vi "Drivetrain Read Encoders.vi"(6 "Reset Encoders":bool) -> (3 "Drivetrain Encoder Values":T1)   [LabVIEW 2016]
uses:
  Common Code/Drivetrain Encoder Values.ctl
  Common Code/Encoder Values.ctl
  Robot Global Data.vi
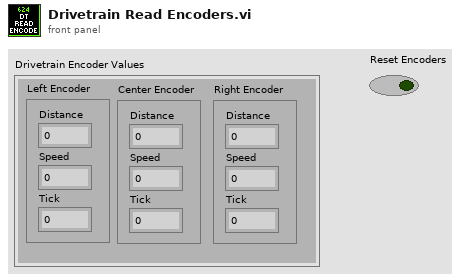
[diagram p1: front panel]
types:
  T1 = typedef "Drivetrain Encoder Values.ctl" = cluster{"Left Encoder":T2, "Center Encoder":T2, "Right Encoder":T2}
  T2 = typedef "Encoder Values.ctl" = cluster{"Distance":dbl, "Speed":dbl, "Tick":dbl}
  T3 = typedef "Dashboard Control Data.ctl" = cluster{"Drivetrain Settings":T4, "Intake Presets ":T6, "Shooter Presets":T7, "Vision Target Packet":T10, "Auton Presets":cluster{"Start Position":dbl}, "Drivetrain Encoder Values":T1, "Drivetrain Encoder Settings":cluster{"Left Tick Constant":dbl, "Right Tick Contant":dbl, "Reset Encoders":bool, "Center Tick Constant":dbl}, "Zero Gyro":bool}
  T4 = typedef "Drivetrain Settings.ctl" = cluster{"Gyro Tolerance":dbl, "Gyro Steer PID Gains":T5, "Y Power Multiplier":dbl, "Turn Power Multiplier":dbl, "Gyro Output":dbl, "Creep Rate":dbl, "Distance Drive PID Gains":T5, "Distance Tolerance":dbl, "Distance Output":dbl, "Strafe Threshold":dbl, "Strafe Correct":bool, "Strafe Corect Tolerance":dbl, "Translate Drive PID Gains":T5, "Strafe Output":dbl, "SC Right":dbl, "SC Left":dbl, "Use Gyro":bool, "Constant Power":bool, "Strafe Power":dbl}
  T5 = typedef "PID Gains.ctl" = cluster{"proportional gain (Kc)":dbl, "integral time (Ti, min)":dbl, "derivative time (Td, min)":dbl}
  T6 = typedef "Intake Presets.ctl" = cluster{"Intake Speed ":dbl, "Outake Speed":dbl, "Current Trip Delay":dbl, "Max Current":dbl}
  T7 = typedef "Shooter Presets.ctl" = cluster{"Key Shot":cluster{"RPM ":dbl, "Hood?":bool}, "Distance Shot":cluster{"RPM":dbl, "Hood?":bool}, "RPM Tolerance":dbl, "Wheel C":dbl, "Vision Shot Presets":T8, "Hopper speed":dbl, "manuel presets":T9}
  T8 = typedef "Vision Shot Presets.ctl" = cluster{"Vision Dist RPM":dbl, "Vision RPM ":dbl, "Vision Dist Hood":bool, "Vision Hood":bool, "Vision Far Dist":dbl, "is we far??":bool}
  T9 = typedef "Manual Shooter Presets.ctl" = cluster{"change delay":dbl}
  T10 = typedef "Vision Target Packet.ctl" = cluster{"Robot Center":dbl, "Center X":dbl, "Center Y":dbl, "Angle":dbl, "Distance":dbl, "Found Target?":bool}
  T11 = typedef "WPI_EncoderDevRef.ctl" = cluster{"DevStatus":errorcluster, "EncoderIndex":T12, "CounterIndex":T13, "DistancePerCount":dbl, "Decoding Type":T14}
  T12 = typedef "FPGA_EncoderIdx.ctl" = enum8{"Enc 0", "Enc 1", "Enc 2", "Enc 3", "Enc 4", "Enc 5", "Enc 6", "Enc 7", "Invalid"}
  T13 = typedef "FPGA_CounterCtrSystemIndex.ctl" = enum8{"Ctr 0", "Ctr 1", "Ctr 2", "Ctr 3", "Ctr 4", "Ctr 5", "Ctr 6", "Ctr 7", "Invalid"}
  T14 = typedef "WPI_EncoderType.ctl" = enum16{"1x", "2x", "4x"}
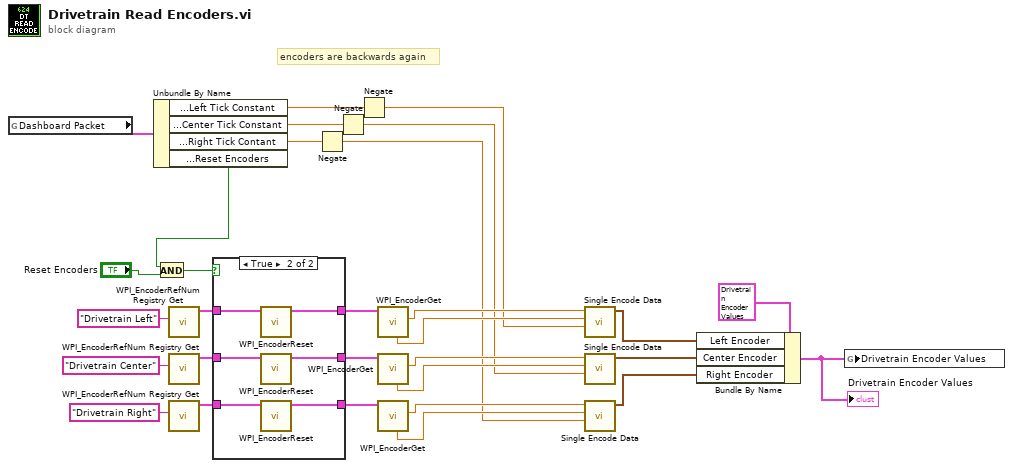
[diagram p0: block diagram]
diagram:
  # "encoders are backwards again"
  n1 = global read "Robot Global Data.vi" "Dashboard Packet"() -> (w13:T3)
  n2 = Unbundle By Name(w13) -> ("Drivetrain Encoder Settings.Left Tick Constant"=w12:dbl, "Drivetrain Encoder Settings.Center Tick Constant"=w11:dbl, "Drivetrain Encoder Settings.Right Tick Contant"=w10:dbl, "Drivetrain Encoder Settings.Reset Encoders"=w1:bool)
  n3 = And(x=w1, y="Reset Encoders") -> (x .and. y?=w2:bool)
  n4 = call <vilib>:"WPI_EncoderRefNum Registry Get.vi"("refnum name"="Drivetrain Left") -> ("EncoderDevRef"=w30:T11)  [unwired: 9 in, 1 out]
  n5 = call <vilib>:"WPI_EncoderRefNum Registry Get.vi"("refnum name"="Drivetrain Center") -> ("EncoderDevRef"=w29:T11)  [unwired: 9 in, 1 out]
  n6 = call <vilib>:"WPI_EncoderRefNum Registry Get.vi"("refnum name"="Drivetrain Right") -> ("EncoderDevRef"=w27:T11)  [unwired: 9 in, 1 out]
  n7 = case shown="True" w2 {
    tunnel: w30 -> [w33 w39]
    tunnel: w29 -> [w32 w38]
    tunnel: w27 -> [w31 w37]
    tunnel: [w33 w36] -> w26
    tunnel: [w32 w35] -> w24
    tunnel: [w31 w34] -> w25
    frame False {
    }
    frame True {
      n8 = call <vilib>:"WPI_EncoderReset.vi"("EncoderDevRef"=w39) -> ("EncoderDevRef"=w36:T11)  [unwired: 9 in, 1 out]
      n9 = call <vilib>:"WPI_EncoderReset.vi"("EncoderDevRef"=w38) -> ("EncoderDevRef"=w35:T11)  [unwired: 9 in, 1 out]
      n10 = call <vilib>:"WPI_EncoderReset.vi"("EncoderDevRef"=w37) -> ("EncoderDevRef"=w34:T11)  [unwired: 9 in, 1 out]
    }
  }
  n11 = Negate(x=w10) -> (-x=w6:dbl)
  n12 = Negate(x=w11) -> (-x=w4:dbl)
  n13 = Negate(x=w12) -> (-x=w5:dbl)
  n14 = call <vilib>:"WPI_EncoderGet.vi"("EncoderDevRef"=w26) -> ("Distance"=w22:dbl, "Rate"=w21:dbl)  [unwired: 5 in, 4 out]
  n15 = call <vilib>:"WPI_EncoderGet.vi"("EncoderDevRef"=w24) -> ("Distance"=w20:dbl, "Rate"=w19:dbl)  [unwired: 5 in, 4 out]
  n16 = call <vilib>:"WPI_EncoderGet.vi"("EncoderDevRef"=w25) -> ("Distance"=w18:dbl, "Rate"=w17:dbl)  [unwired: 5 in, 4 out]
  n17 = call "Single Encode Data.vi"("Tick Constant"=w5, "Rate"=w21, "Distance"=w22) -> ("Encoder Values"=w16:T2)  [unwired: 8 in]
  n18 = call "Single Encode Data.vi"("Tick Constant"=w4, "Rate"=w19, "Distance"=w20) -> ("Encoder Values"=w15:T2)  [unwired: 8 in]
  n19 = call "Single Encode Data.vi"("Tick Constant"=w6, "Rate"=w17, "Distance"=w18) -> ("Encoder Values"=w14:T2)  [unwired: 8 in]
  n20 = Bundle By Name(cluster=T1 {"Left Encoder"={"Distance"=0.0, "Speed"=0.0, "Tick"=0.0}, "Center Encoder"={"Distance"=0.0, "Speed"=0.0, "Tick"=0.0}, "Right Encoder"={"Distance"=0.0, "Speed"=0.0, "Tick"=0.0}} ("Drivetrain Encoder Values"), "Left Encoder"=w16, "Center Encoder"=w15, "Right Encoder"=w14) -> (w9:T1)
  "Drivetrain Encoder Values" <- w9
  n21 = global write "Robot Global Data.vi" "Drivetrain Encoder Values"(w9) -> ()
